vi "GE 5565PIORC.Memory.Read from DMA Block.vi"   [LabVIEW 2016, in "GE 5565PIORC.lvclass"]
doc: "Reads <B>count</B> elements from the provided <B>Block Descriptor</B> into a newly allocated <B>data</B> array."
uses:
  GE 5565PIORC.lvclass
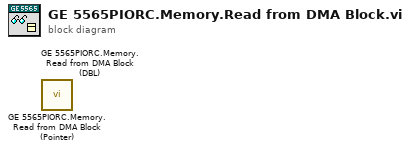
[diagram p0: block diagram]
diagram:
  n1 = call "GE 5565PIORC.Memory.Read from DMA Block (Pointer).vi"() -> ()  [unwired: 8 in, 4 out]
  n2 = call "GE 5565PIORC.Memory.Read from DMA Block (DBL).vi"() -> ()  [unwired: 8 in, 4 out]
